vi "Init Bfr Rx - Create Option Channels.vi"(5 "External Buffer":bool, 6 "Rx Buffer Option":T4, 7 "Packet Name":string, 8 "error in (no error)":errorcluster, 11 "Data Access":refnum<class "Data Access Engine.lvclass">) -> (0 "error out":errorcluster, 3 "Buffer Options":cluster{"Ping Pong":T1})   [LabVIEW 2019, in "UDP-Custom-Device Engine.lvlib"]
uses:
  UDP-Custom-Device Engine.lvlib
  <vilib>/NI/NIVS Inline Async API/_Data Access Engine/Data Access Engine/Data Access Engine.lvclass
  Shared/Types/Shared - Receive Buffer Options.ctl
  Types/Engine - Buffered Rx Ping Pong Channels.ctl
  <vilib>/NI/NIVS Inline Async API/_Data Access Engine/Data Access Engine/Types/Read.DVR.ctl
  <vilib>/NI/NIVS Inline Async API/_Data Access Engine/Access Type Classes/Read/Read.lvclass
  <vilib>/NI/NIVS Inline Async API/_Data Access Engine/Data Access Engine/Types/Write.DVR.ctl
  <vilib>/NI/NIVS Inline Async API/_Data Access Engine/Access Type Classes/Write/Write.lvclass
  <vilib>/NI/NIVS Inline Async API/_Data Access Engine/Data Access Engine/Methods/Read.Lookup.vi
  <vilib>/NI/NIVS Inline Async API/_Data Access Engine/Data Access Engine/Methods/Write.Lookup.vi
  Shared/UDP-Custom-Device Shared.lvlib
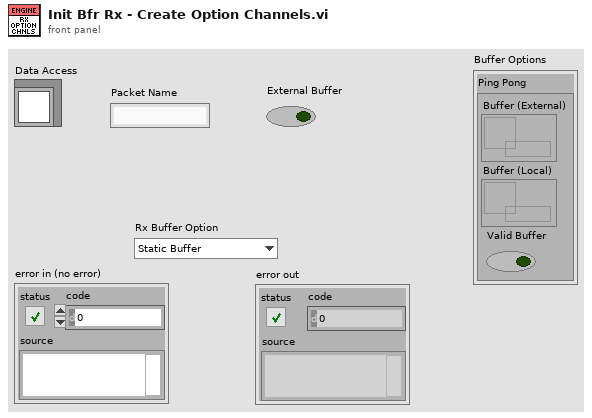
[diagram p1: front panel]
types:
  T1 = typedef "UDP-Custom-Device Engine.lvlib/Engine - Buffered Rx Ping Pong Channels.ctl" = cluster{"Buffer (External)":T2, "Buffer (Local)":T3, "Valid Buffer":bool}
  T2 = typedef "Data Access Engine.lvlib/Data Access Engine.lvclass/Read.DVR.ctl" = refnum<data-value>
  T3 = typedef "Data Access Engine.lvlib/Data Access Engine.lvclass/Write.DVR.ctl" = refnum<data-value>
  T4 = typedef "UDP-Custom-Device Shared.lvlib/Shared - Receive Buffer Options.ctl" = enum16{"Static Buffer", "Circular Buffer", "Circular Buffer + Size", "Internal Cache", "Internal Cache + Size", "Ping Pong", "Ping Pong + Size"}
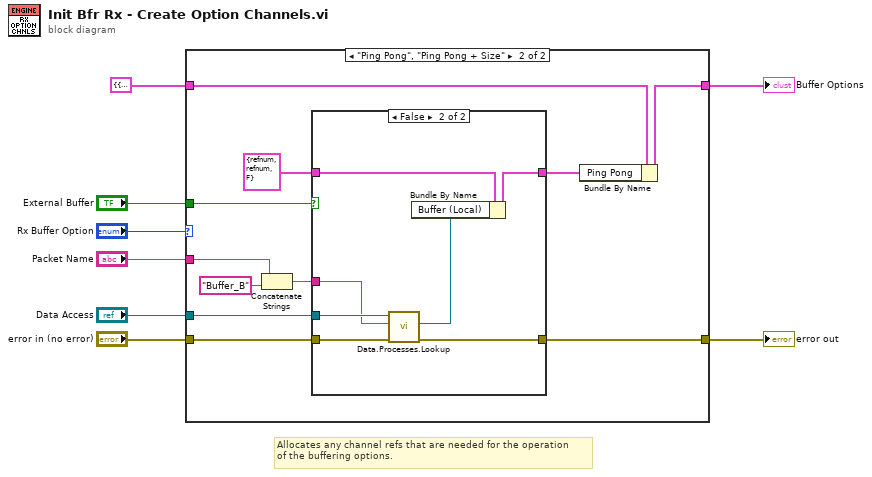
[diagram p0: block diagram]
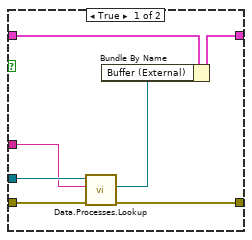
[diagram p3: hidden frame]
diagram:
  # "Allocates any channel refs that are needed for the operation\nof the buffering options."
  n1 = case shown="\"Ping Pong\", \"Ping Pong + Size\"" "Rx Buffer Option" {
    tunnel: "External Buffer" -> [_ w19]
    tunnel: "Packet Name" -> [_ w17]
    tunnel: "Data Access" -> [_ w21]
    tunnel: "error in (no error)" -> [w10 w20]
    tunnel: [w10 w15] -> w3
    tunnel: [w9 w11] -> w2
    tunnel: cluster{"Ping Pong":T1} {"Ping Pong"={"Buffer (External)"=refnum, "Buffer (Local)"=refnum, "Valid Buffer"=FALSE}} ("Buffer Options") -> [w9 w13]
    frame Default {
    }
    frame "Ping Pong", "Ping Pong + Size" {
      n2 = Concatenate Strings(w17, "Buffer_B" ("Item GUID")) -> (w16:string)
      n3 = case shown="False" w19 {
        tunnel: w21 -> [w28 w35]
        tunnel: w20 -> [w27 w34]
        tunnel: w16 -> [w26 w33]
        tunnel: [w25 w32] -> w15
        tunnel: T1 {"Buffer (External)"=refnum, "Buffer (Local)"=refnum, "Valid Buffer"=FALSE} ("Ping Pong") -> [w24 w31]
        tunnel: [w22 w29] -> w12
        frame True {
          n4 = call-poly <vilib>:"Data.Processes.Lookup.vi"("error in (no error)"=w27, "Name"=w26, "Data Access API in"=w28) -> ("error out"=w25:errorcluster, "Ref"=w23:T2)  [unwired: 5 in, 2 out]
          n5 = Bundle By Name(cluster=w24, "Buffer (External)"=w23) -> (w22:T1)
        }
        frame False {
          n6 = call-poly <vilib>:"Data.Processes.Lookup.vi"("error in (no error)"=w34, "Name"=w33, "Data Access API in"=w35) -> ("error out"=w32:errorcluster, "Ref"=w30:T3)  [unwired: 5 in, 2 out]
          n7 = Bundle By Name(cluster=w31, "Buffer (Local)"=w30) -> (w29:T1)
        }
      }
      n8 = Bundle By Name(cluster=w13, "Ping Pong"=w12) -> (w11:cluster{"Ping Pong":T1})
    }
  }
  "error out" <- w3
  "Buffer Options" <- w2
